vi "hla_outgoing_queue_instance_6.vi"(2 "InteractionRoot.C2WInteractionRoot.FederateResignInteraction":T1, 5 "error in (no error)":errorcluster) -> (19 "error out":errorcluster)   [LabVIEW 2016]
uses:
  objects_and_interfaces/InteractionRoot.C2WInteractionRoot.FederateResignInteraction.ctl
  utilities/runtime/support/controls/queue_assistant_actions.ctl
  utilities/runtime/support/controls/entity.ctl
  utilities/runtime/support/controls/entity_type.ctl
  utilities/runtime/support/controls/queue_type.ctl
  <vilib>/Utility/Data Type/NI_Data Type.lvlib
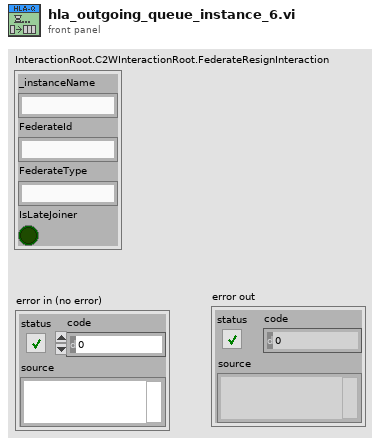
[diagram p1: front panel]
types:
  T1 = typedef "InteractionRoot.C2WInteractionRoot.FederateResignInteraction.ctl" = cluster{"_instanceName":string, "FederateId":string, "FederateType":string, "IsLateJoiner":bool}
  T2 = typedef "queue_type.ctl" = enum16{"all", "dostep", "entities_incoming", "entities_outoing", "response"}
  T3 = typedef "entity.ctl" = cluster{"type":T4, "classPath":string, "params":string[][], "instanceName":string}
  T4 = typedef "entity_type.ctl" = string
  T5 = typedef "queue_assistant_actions.ctl" = enum16{"--- unused ---", "bulk_enq_ahead", "bulk_enq_behind", "destroy", "empty?", "enq_ahead", "enq_behind", "flush", "get_queues", "init"}
  T6 = typedef "NI_Data Type.lvlib/Data Type.ctl" = enum8{"Invalid Type", "Void", "I8", "I16", "I32", "I64", "U8", "U16", "U32", "U64", "Single Float", "Double Float", "Extended Float", "Single Complex", "Double Complex", "Extended Complex", "Enum U8", "Enum U16", "Enum U32", "Enum U64", "Single Float With Unit", "Double Float With Unit", "Extended Float With Unit", "Single Complex with Unit", "Double Complex with Unit", "Extended Complex with Unit", "Boolean", "String", "Path", "Picture", "Tag", "Array", "Cluster", "Variant", "LV Variant", "Waveform", "Timestamp", "Digital Waveform", "Digital Data", "ExpressData", "Refnum", "External Data", "VI", "Poly VI", "LabVIEW Class Instance", "Fixed Point"}
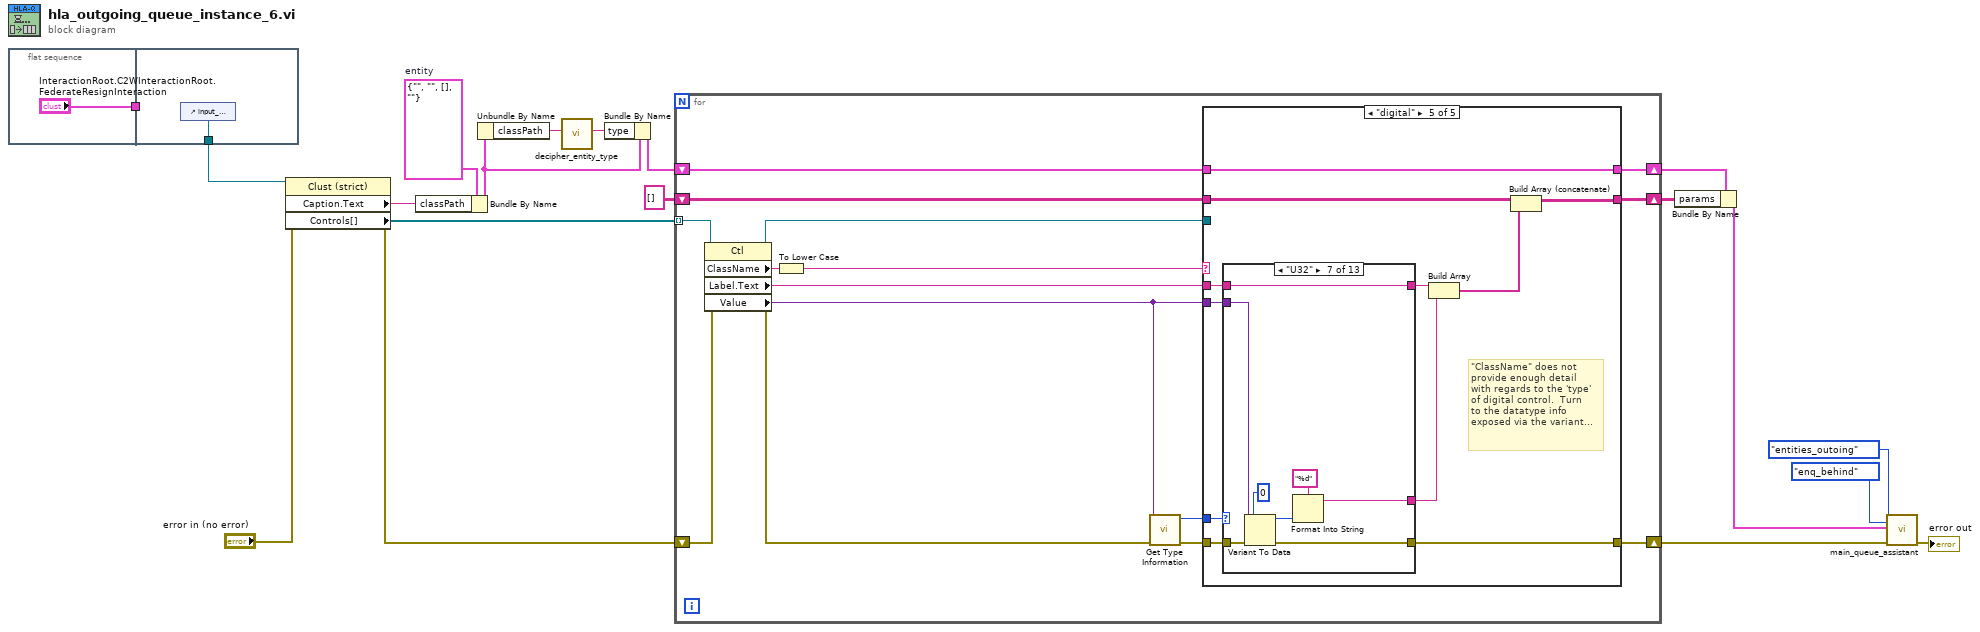
[diagram p0: block diagram]
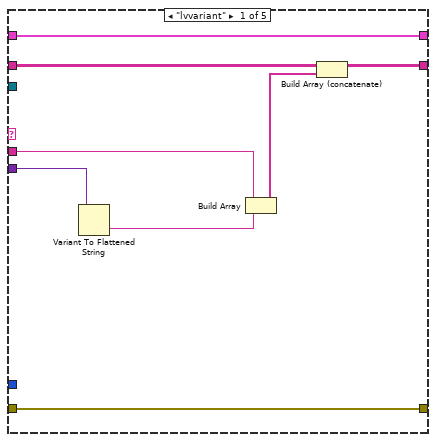
[diagram p2: hidden frame]
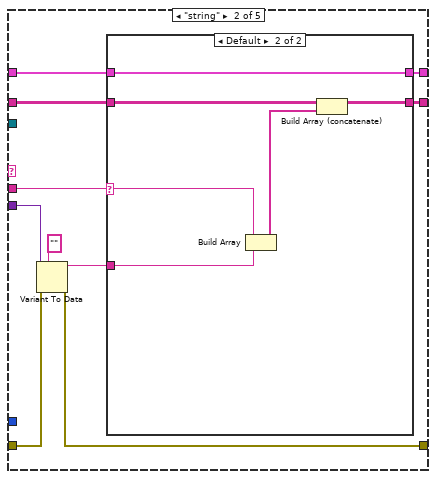
[diagram p3: hidden frame]
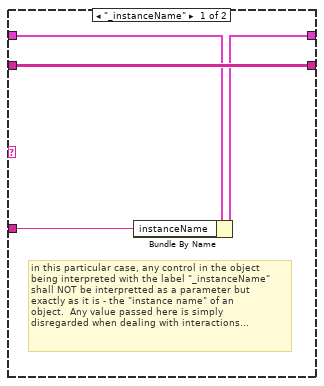
[diagram p4: hidden frame]
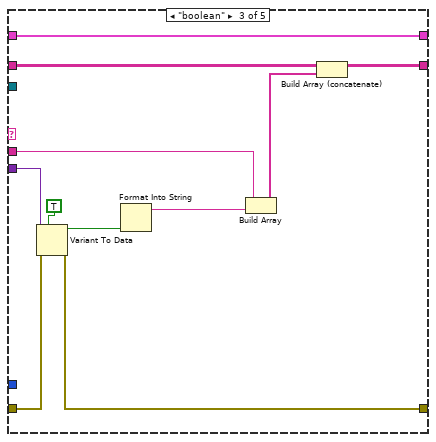
[diagram p5: hidden frame]
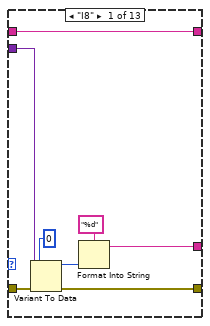
[diagram p7: hidden frame]
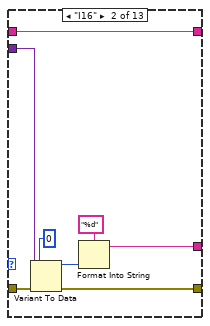
[diagram p8: hidden frame]
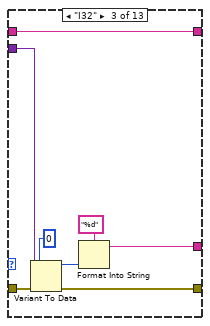
[diagram p9: hidden frame]
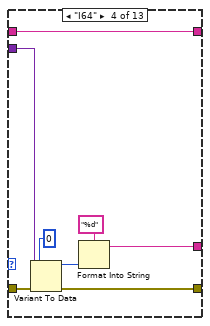
[diagram p10: hidden frame]
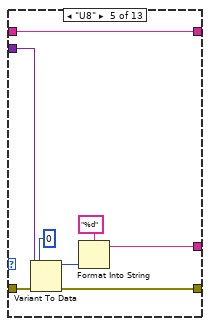
[diagram p11: hidden frame]
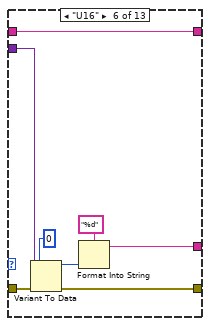
[diagram p12: hidden frame]
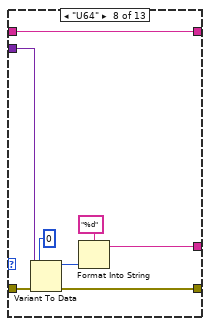
[diagram p13: hidden frame]
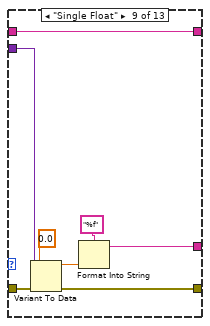
[diagram p14: hidden frame]
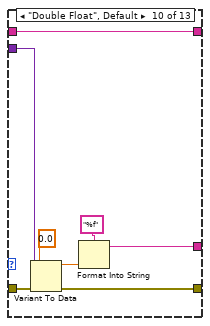
[diagram p15: hidden frame]
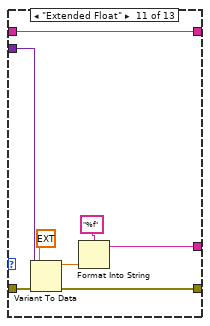
[diagram p16: hidden frame]
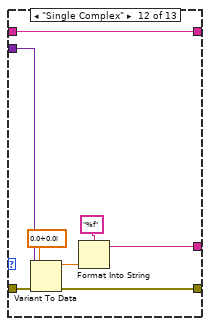
[diagram p17: hidden frame]
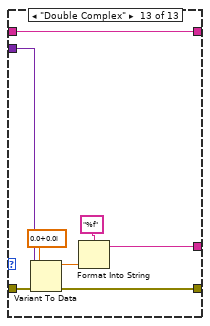
[diagram p18: hidden frame]
diagram:
  w16 = T3 {"type"="", "classPath"="", "params"=[], "instanceName"=""}  # entity
  n1 = flat-sequence {
    tunnel: ["InteractionRoot.C2WInteractionRoot.FederateResignInteraction"] -> w9
    tunnel: [w21] -> w10
    tunnel: w9 -> [_]
    frame #0 {
    }
    frame #1 {
      n2 = control-ref of="input_cluster"() -> (w21:refnum<vi>)
    }
  }
  n3 = property class="Clust (strict)"(reference=w10, error in="error in (no error)") -> (error out=w18:errorcluster, "Caption.Text"=w15:string, "Controls[]"=w17:refnum<vi>[])  [unwired: 1 out]
  n4 = Bundle By Name(cluster=w16, "classPath"=w15) -> (w8:T3)
  n5 = Unbundle By Name(w8) -> ("classPath"=w7:string)
  n6 = call "decipher_entity_type.vi"("classpath (fully qualified)"=w7) -> ("entity_type (out)"=w6:T4)  [unwired: 10 in]
  n7 = Bundle By Name(cluster=w8, "type"=w6) -> (w2:T3)
  n8 = for {
    tunnel: w17 -> [w35] mode=indexing
    shift-right: [w31] -> w11
    shift-left: w18 -> [w36]
    shift-right: [w24] -> w13
    shift-left: string[][] [] -> [w30]
    shift-right: [w22] -> w1
    shift-left: w2 -> [w23]
    n9 = property class="Ctl"(reference=w35, error in=w36) -> (reference out=w33:refnum<vi>, error out=w27:errorcluster, "ClassName"=w34:string, "Label.Text"=w29:string, "Value"=w28:variant)
    n10 = To Lower Case(string=w34) -> (all lower case string=w32:string)
    n11 = call <vilib>:"Get Type Information.vi"("error in (no error)"=w27, "Variant"=w28) -> ("error out"=w26:errorcluster, "Type"=w25:T6)  [unwired: 5 in, 3 out]
    n12 = case shown="\"digital\"" w32 {
      tunnel: w33 -> [_ _ _ _ _]
      tunnel: w26 -> [w42 w51 w71 w78 w89]
      tunnel: [w42 w50 w70 w78 w84] -> w31
      tunnel: w30 -> [w43 w54 w74 w77 w88]
      tunnel: w29 -> [w39 w47 w68 _ w87]
      tunnel: w28 -> [w44 w53 w73 _ w85]
      tunnel: [w38 w49 w66 w77 w80] -> w24
      tunnel: w25 -> [_ _ _ _ w86]
      tunnel: w23 -> [w37 w46 w65 w76 w79]
      tunnel: [w37 w45 w65 w76 w79] -> w22
      frame "lvvariant" {
        n13 = Variant To Flattened String(Variant=w44) -> (data string=w41:string)  [unwired: 1 out]
        n14 = Build Array(w39, w41) -> (w40:string[])
        n15 = Build Array (concatenate)(w43, w40) -> (w38:string[][])
      }
      frame "string" {
        n16 = Variant To Data(error in=w51, type="", Variant=w53) -> (data=w48:string, error out=w50:errorcluster)
        n17 = case shown="Default" w47 {
          selector: w47 -> [_ w60]
          tunnel: w54 -> [w58 w64]
          tunnel: [w58 w63] -> w49
          tunnel: w48 -> [w56 w62]
          tunnel: w46 -> [w57 w59]
          tunnel: [w55 w59] -> w45
          frame "_instanceName" {
            # "in this particular case, any control in the object\nbeing interpreted with the label \"_instanceName\"\nshall NOT be interpretted as a parameter but\nexactly as it is - the \"instance name\" of an \nobject.  Any value passed here is simply \ndisregarded when dealing with interactions..."
            n18 = Bundle By Name(cluster=w57, "instanceName"=w56) -> (w55:T3)
          }
          frame Default {
            n19 = Build Array(w60, w62) -> (w61:string[])
            n20 = Build Array (concatenate)(w64, w61) -> (w63:string[][])
          }
        }
      }
      frame "boolean" {
        n21 = Variant To Data(error in=w71, type=TRUE, Variant=w73) -> (data=w69:bool, error out=w70:errorcluster)
        n22 = Format Into String(w69) -> (resulting string=w67:string)  [unwired: 3 in, 1 out]
        n23 = Build Array(w68, w67) -> (w75:string[])
        n24 = Build Array (concatenate)(w74, w75) -> (w66:string[][])
      }
      frame Default {
        # "if the ClassName is undefined"
      }
      frame "digital" {
        # "\"ClassName\" does not\nprovide enough detail\nwith regards to the 'type'\nof digital control.  Turn\nto the datatype info\nexposed via the variant..."
        n25 = case shown="\"U32\"" w86 {
          tunnel: w89 -> [w97 w105 w113 w121 w129 w137 w145 w153 w161 w169 w177 w185 w193]
          tunnel: w87 -> [w92 w100 w108 w116 w124 w132 w140 w148 w156 w164 w172 w180 w188]
          tunnel: w85 -> [w96 w104 w112 w120 w128 w136 w144 w152 w160 w168 w176 w184 w192]
          tunnel: [w92 w100 w108 w116 w124 w132 w140 w148 w156 w164 w172 w180 w188] -> w83
          tunnel: [w91 w99 w107 w115 w123 w131 w139 w147 w155 w163 w171 w179 w187] -> w82
          tunnel: [w90 w98 w106 w114 w122 w130 w138 w146 w154 w162 w170 w178 w186] -> w84
          frame "I8" {
            n26 = Variant To Data(error in=w97, type=i8 0, Variant=w96) -> (data=w94:i8, error out=w90:errorcluster)
            n27 = Format Into String(format string="%d", w94) -> (resulting string=w91:string)  [unwired: 2 in, 1 out]
          }
          frame "I16" {
            n28 = Variant To Data(error in=w105, type=i16 0, Variant=w104) -> (data=w102:i16, error out=w98:errorcluster)
            n29 = Format Into String(format string="%d", w102) -> (resulting string=w99:string)  [unwired: 2 in, 1 out]
          }
          frame "I32" {
            n30 = Variant To Data(error in=w113, type=0, Variant=w112) -> (data=w110:i32, error out=w106:errorcluster)
            n31 = Format Into String(format string="%d", w110) -> (resulting string=w107:string)  [unwired: 2 in, 1 out]
          }
          frame "I64" {
            n32 = Variant To Data(error in=w121, type=i64 0, Variant=w120) -> (data=w118:i64, error out=w114:errorcluster)
            n33 = Format Into String(format string="%d", w118) -> (resulting string=w115:string)  [unwired: 2 in, 1 out]
          }
          frame "U8" {
            n34 = Variant To Data(error in=w129, type=u8 0, Variant=w128) -> (data=w126:u8, error out=w122:errorcluster)
            n35 = Format Into String(format string="%d", w126) -> (resulting string=w123:string)  [unwired: 2 in, 1 out]
          }
          frame "U16" {
            n36 = Variant To Data(error in=w137, type=u16 0, Variant=w136) -> (data=w134:u16, error out=w130:errorcluster)
            n37 = Format Into String(format string="%d", w134) -> (resulting string=w131:string)  [unwired: 2 in, 1 out]
          }
          frame "U32" {
            n38 = Variant To Data(error in=w145, type=u32 0, Variant=w144) -> (data=w142:u32, error out=w138:errorcluster)
            n39 = Format Into String(format string="%d", w142) -> (resulting string=w139:string)  [unwired: 2 in, 1 out]
          }
          frame "U64" {
            n40 = Variant To Data(error in=w153, type=u64 0, Variant=w152) -> (data=w150:u64, error out=w146:errorcluster)
            n41 = Format Into String(format string="%d", w150) -> (resulting string=w147:string)  [unwired: 2 in, 1 out]
          }
          frame "Single Float" {
            n42 = Variant To Data(error in=w161, type=sgl 0.0, Variant=w160) -> (data=w158:sgl, error out=w154:errorcluster)
            n43 = Format Into String(format string="%f", w158) -> (resulting string=w155:string)  [unwired: 2 in, 1 out]
          }
          frame "Double Float", Default {
            n44 = Variant To Data(error in=w169, type=0.0, Variant=w168) -> (data=w166:dbl, error out=w162:errorcluster)
            n45 = Format Into String(format string="%f", w166) -> (resulting string=w163:string)  [unwired: 2 in, 1 out]
          }
          frame "Extended Float" {
            n46 = Variant To Data(error in=w177, type=ext 0.0, Variant=w176) -> (data=w174:ext, error out=w170:errorcluster)
            n47 = Format Into String(format string="%f", w174) -> (resulting string=w171:string)  [unwired: 2 in, 1 out]
          }
          frame "Single Complex" {
            n48 = Variant To Data(error in=w185, type=csg 0.0+0.0i, Variant=w184) -> (data=w182:csg, error out=w178:errorcluster)
            n49 = Format Into String(format string="%f", w182) -> (resulting string=w179:string)  [unwired: 2 in, 1 out]
          }
          frame "Double Complex" {
            n50 = Variant To Data(error in=w193, type=cdb 0.0+0.0i, Variant=w192) -> (data=w190:cdb, error out=w186:errorcluster)
            n51 = Format Into String(format string="%f", w190) -> (resulting string=w187:string)  [unwired: 2 in, 1 out]
          }
        }
        n52 = Build Array(w83, w82) -> (w81:string[])
        n53 = Build Array (concatenate)(w88, w81) -> (w80:string[][])
      }
    }
  }
  n54 = Bundle By Name(cluster=w1, "params"=w13) -> (w3:T3)
  n55 = call "main_queue_assistant.vi"("queue_type (def=all)"=queue_type."entities_outoing", "action (enq_behind = def)"=queue_assistant_actions."enq_behind" ("queue_action (enq_behind = def)"), "entity"=w3, "error in (no error)"=w11) -> ("error out"=→"error out":errorcluster)  [unwired: 13 in, 2 out]
